vi "test.vi"() -> ()   [LabVIEW 2017]
uses:
  Downloads/axiocam_ng_sdk_1.78/AxiocamSDK/api/lib/axcam64.dll
panel:
  out "return type":i32
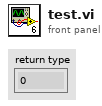
[diagram p1: front panel]
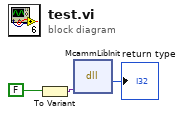
[diagram p0: block diagram]
diagram:
  n1 = To Variant(anything=FALSE) -> (Variant=w3:variant)
  n2 = dll-call lib="C:/Users/OmerLab/Downloads/axiocam_ng_sdk_1.78/AxiocamSDK/api/lib/axcam64.dll" fn="McammLibInit"("arg1"=w3) -> ("return type"=→"return type":i32)  [unwired: 4 in, 2 out]
